vi "JSON Minify.vi"(8 "error in":errorcluster, 10 "JSON String":string) -> (0 "error out":errorcluster, 2 "JSON Minified":string)   [LabVIEW 2020]
doc: "This VI allows minifying the JSON prior to parsing to avoid any errors.\nThe algorithm is ported from https://github.com/getify/JSON.minify.\n---\nAuthor: Felipe P. Silva"
uses:
  <vilib>/regexp/Match Regular Expression.xnode
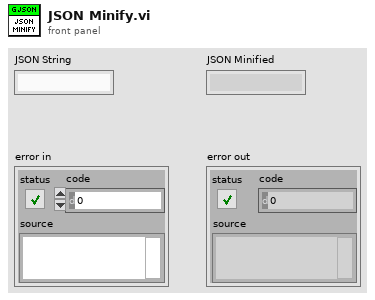
[diagram p1: front panel]
types:
  T1 = cluster{"in_multiline_comment":bool, "in_singleline_comment":bool, "in_string":bool, "new_str":string[], "from":i32, "lc":string, "rc":string}
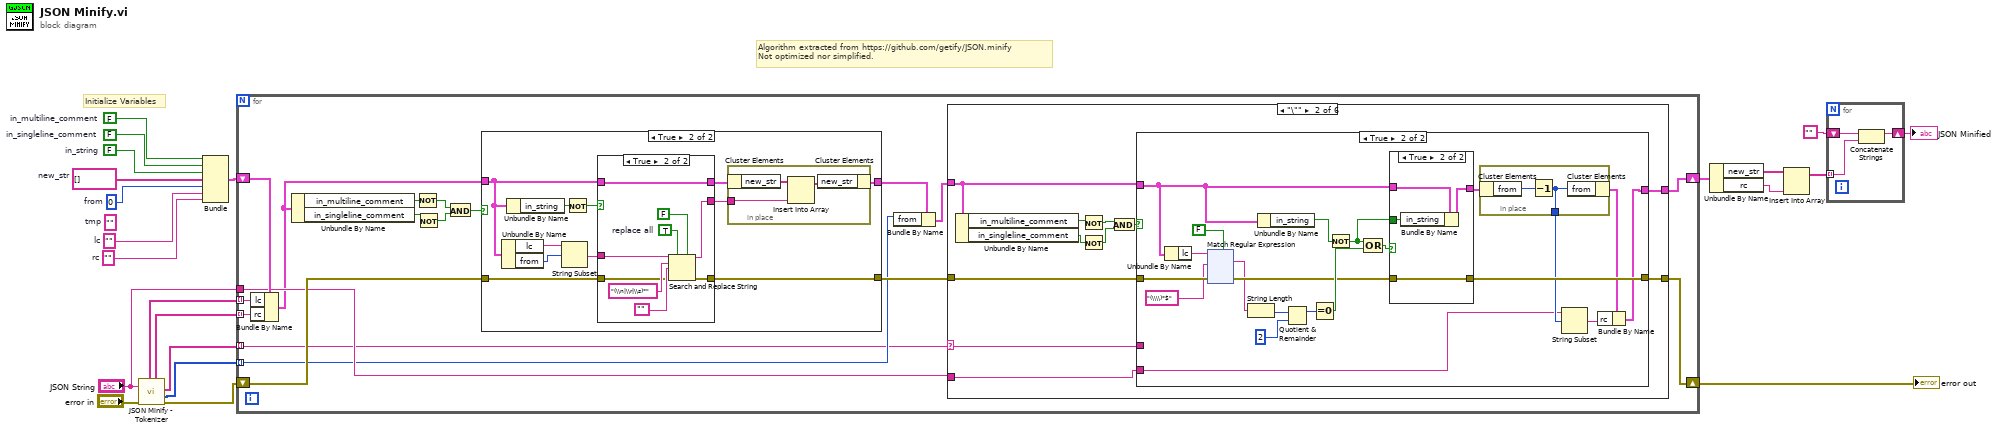
[diagram p0: block diagram]
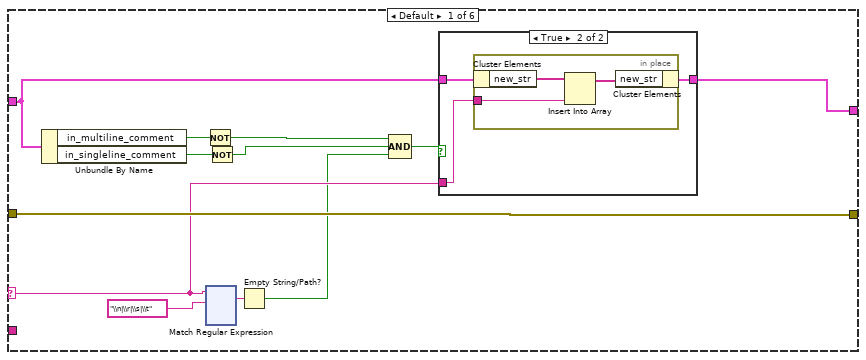
[diagram p2: hidden frame]
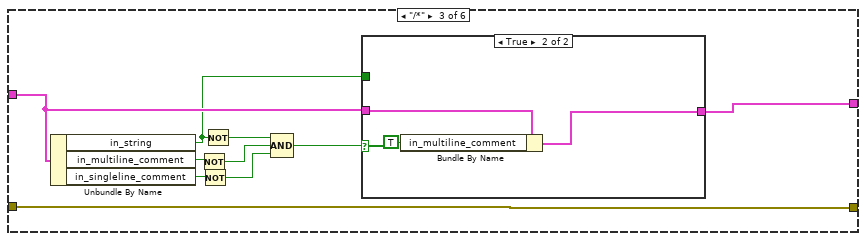
[diagram p6: hidden frame]
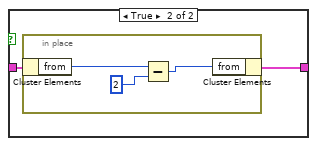
[diagram p8: hidden frame]
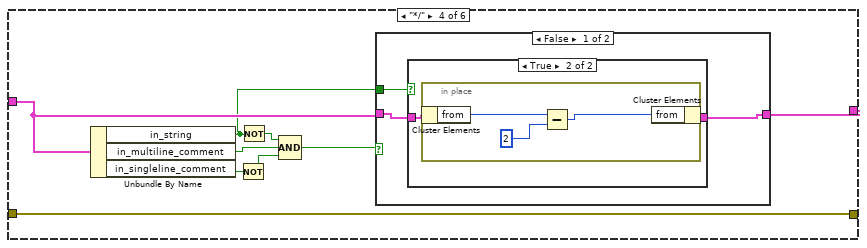
[diagram p9: hidden frame]
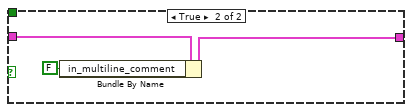
[diagram p11: hidden frame]
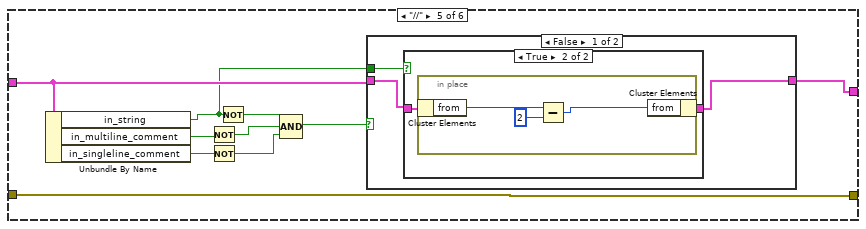
[diagram p12: hidden frame]
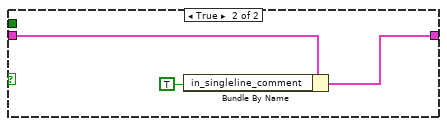
[diagram p14: hidden frame]
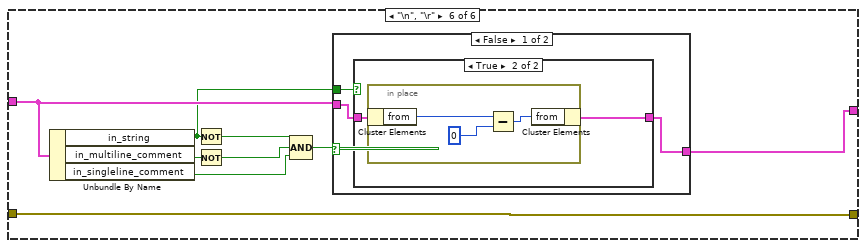
[diagram p15: hidden frame]
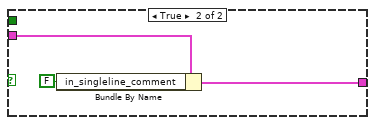
[diagram p17: hidden frame]
diagram:
  w12 = ""  # rc
  w13 = ""  # lc
  (unwired) ""  # tmp
  w19 = string[] []  # new_str
  w20 = FALSE  # in_string
  w21 = FALSE  # in_singleline_comment
  w22 = FALSE  # in_multiline_comment
  w17 = 0  # from
  # "Algorithm extracted from https://github.com/getify/JSON.minify\nNot optimized nor simplified."
  # "Initialize Variables"
  n1 = call "JSON Minify - Tokenizer.vi"("error in (no error)"="error in", "JSON String"="JSON String") -> ("error out"=w6:errorcluster, "offset past"=w5:i32[], "matches"=w4:string[], "Right Context"=w2:string[], "Left Context"=w3:string[])  [unwired: 5 in]
  n2 = Bundle("in_multiline_comment"=w22, "in_singleline_comment"=w21, "in_string"=w20, "new_str"=w19, "from"=w17, "lc"=w13, "rc"=w12) -> (w16:T1)  [unwired: 1 in]
  n3 = for {
    shift-right: [w29] -> w18
    shift-left: w6 -> [w35]
    shift-right: [w28] -> w11
    shift-left: w16 -> [w36]
    tunnel: w4 -> [w26] mode=indexing
    tunnel: "JSON String" -> [w32]
    tunnel: w5 -> [w27] mode=indexing
    tunnel: w3 -> [w24] mode=indexing
    tunnel: w2 -> [w23] mode=indexing
    n4 = Bundle By Name(cluster=w36, "lc"=w24, "rc"=w23) -> (w25:T1)
    n5 = Unbundle By Name(w25) -> ("in_multiline_comment"=w31:bool, "in_singleline_comment"=w30:bool)
    n6 = Not(x=w31) -> (.not. x?=w40:bool)
    n7 = Not(x=w30) -> (.not. x?=w39:bool)
    n8 = And(x=w40, y=w39) -> (x .and. y?=w37:bool)
    n9 = case shown="True" w37 {
      tunnel: w25 -> [w417 w421]
      tunnel: [w417 w425] -> w34
      tunnel: [w416 w428] -> w38
      tunnel: w35 -> [w416 w418]
      frame False {
      }
      frame True {
        n10 = Unbundle By Name(w421) -> ("lc"=w424:string, "from"=w423:i32)
        n11 = Unbundle By Name(w421) -> ("in_string"=w420:bool)
        n12 = String Subset(string=w424, offset (0)=w423) -> (substring=w422:string)  [unwired: 1 in]
        n13 = Not(x=w420) -> (.not. x?=w419:bool)
        n14 = case shown="True" w419 {
          tunnel: [w433 w443] -> w428
          tunnel: w421 -> [w434 w440]
          tunnel: [w434 w440] -> w426
          tunnel: [w432 w441] -> w427
          tunnel: w422 -> [w432 w438]
          tunnel: w418 -> [w433 w437]
          frame False {
          }
          frame True {
            w436 = TRUE  # replace all
            n15 = Search and Replace String(replace all?=w436, multiline?=FALSE ("multiline? (F)"), input string=w438, search string="(\\n|\\r|\\s)*", replace string="" ("replace string (\"\")"), error in=w437) -> (result string=w441:string, error out=w443:errorcluster)  [unwired: 2 in, 2 out]
          }
        }
        n16 = in-place {
          in-place-border: w427 -> [w430]
          n17 = in-place-cluster #1(w426) -> ("new_str"=w429:string[])
          n18 = Insert Into Array(array=w429, new element=w430) -> (w431:string[])  [unwired: 1 in]
          n19 = in-place-cluster #1("new_str"=w431) -> (w425:T1)
        }
      }
    }
    n20 = Bundle By Name(cluster=w34, "from"=w27) -> (w33:T1)
    n21 = case shown="\"\\\"\"" w26 {
      selector: w26 -> [w42 w175 _ _ _ _]
      tunnel: w33 -> [w51 w180 w338 w359 w381 w402]
      tunnel: [w50 w174 w336 w358 w380 w401] -> w28
      tunnel: w38 -> [w52 w183 w339 w360 w382 w403]
      tunnel: [w52 w184 w339 w360 w382 w403] -> w29
      tunnel: w32 -> [_ w176 _ _ _ _]
      frame Default {
        n22 = Unbundle By Name(w51) -> ("in_multiline_comment"=w46:bool, "in_singleline_comment"=w45:bool)
        n23 = Not(x=w46) -> (.not. x?=w49:bool)
        n24 = xnode "Match Regular Expression"("input string"=w42, "regular expression"="\\n|\\r|\\s|\\t") -> ("whole match"=w43:string)  [unwired: 4 in, 4 out]
        n25 = Not(x=w45) -> (.not. x?=w48:bool)
        n26 = Empty String/Path?(string/path=w43) -> (empty?=w41:bool)
        n27 = Compound Arithmetic op=AND(w49, w48, w41) -> (w47:bool)
        n28 = case shown="True" w47 {
          tunnel: w51 -> [w53 w56]
          tunnel: [w53 w55] -> w50
          tunnel: w42 -> [_ w54]
          frame False {
          }
          frame True {
            n29 = in-place {
              in-place-border: w54 -> [w57]
              n30 = in-place-cluster #2(w56) -> ("new_str"=w58:string[])
              n31 = Insert Into Array(array=w58, new element=w57) -> (w59:string[])  [unwired: 1 in]
              n32 = in-place-cluster #2("new_str"=w59) -> (w55:T1)
            }
          }
        }
      }
      frame "\"" {
        n33 = Unbundle By Name(w180) -> ("in_multiline_comment"=w178:bool, "in_singleline_comment"=w177:bool)
        n34 = Not(x=w178) -> (.not. x?=w181:bool)
        n35 = Not(x=w177) -> (.not. x?=w182:bool)
        n36 = And(x=w181, y=w182) -> (x .and. y?=w179:bool)
        n37 = case shown="True" w179 {
          tunnel: [w185 w207] -> w184
          tunnel: w183 -> [w185 w194]
          tunnel: [w186 w198] -> w174
          tunnel: w180 -> [w186 w199]
          tunnel: w176 -> [_ w196]
          tunnel: w175 -> [_ _]
          frame False {
          }
          frame True {
            n38 = Unbundle By Name(w199) -> ("lc"=w192:string)
            n39 = xnode "Match Regular Expression"("input string"=w192, "regular expression"="(\\\\)*$", "error in"=w194, "multiline? (F)"=FALSE) -> ("whole match"=w189:string, "error out"=w193:errorcluster)  [unwired: 2 in, 3 out]
            n40 = String Length(string=w189) -> (length=w190:i32)
            n41 = Unbundle By Name(w199) -> ("in_string"=w201:bool)
            n42 = Quotient & Remainder(x=w190, y=2) -> (x-y*floor(x/y)=w187:i32)  [unwired: 1 out]
            n43 = Equal To 0?(x=w187) -> (x = 0?=w202:bool)
            n44 = Not(x=w201) -> (.not. x?=w204:bool)
            n45 = Compound Arithmetic op=OR(w204, w202) -> (w205:bool)
            n46 = case shown="True" w205 {
              tunnel: [w210 w215] -> w207
              tunnel: w193 -> [w210 w215]
              tunnel: [w211 w213] -> w206
              tunnel: w199 -> [w211 w214]
              tunnel: w204 -> [_ w212]
              frame False {
              }
              frame True {
                n47 = Bundle By Name(cluster=w214, "in_string"=w212) -> (w213:T1)
              }
            }
            n48 = in-place {
              in-place-border: [w208] -> w197
              n49 = in-place-cluster #3(w206) -> ("from"=w209:i32)
              n50 = Decrement(x=w209) -> (x-1=w208:i32)
              n51 = in-place-cluster #3("from"=w208) -> (w200:T1)
            }
            n52 = String Subset(string=w196, offset (0)=w197) -> (substring=w195:string)  [unwired: 1 in]
            n53 = Bundle By Name(cluster=w200, "rc"=w195) -> (w198:T1)
          }
        }
      }
      frame "/*" {
        n54 = Unbundle By Name(w338) -> ("in_string"=w330:bool, "in_multiline_comment"=w335:bool, "in_singleline_comment"=w334:bool)
        n55 = Not(x=w335) -> (.not. x?=w332:bool)
        n56 = Not(x=w334) -> (.not. x?=w333:bool)
        n57 = Not(x=w330) -> (.not. x?=w331:bool)
        n58 = Compound Arithmetic op=AND(w331, w332, w333) -> (w337:bool)
        n59 = case shown="True" w337 {
          tunnel: w338 -> [w342 w351]
          tunnel: [w341 w350] -> w336
          tunnel: w330 -> [w340 _]
          frame False {
            n60 = case shown="False" w340 {
              tunnel: w342 -> [w343 w345]
              tunnel: [w343 w344] -> w341
              frame False {
              }
              frame True {
                n61 = in-place {
                  n62 = in-place-cluster #4(w345) -> ("from"=w348:i32)
                  n63 = Subtract(x=w348, y=2) -> (x-y=w347:i32)
                  n64 = in-place-cluster #4("from"=w347) -> (w344:T1)
                }
              }
            }
          }
          frame True {
            n65 = Bundle By Name(cluster=w351, "in_multiline_comment"=TRUE) -> (w350:T1)
          }
        }
      }
      frame "*/" {
        n66 = Unbundle By Name(w359) -> ("in_string"=w352:bool, "in_multiline_comment"=w354:bool, "in_singleline_comment"=w353:bool)
        n67 = Not(x=w353) -> (.not. x?=w356:bool)
        n68 = Not(x=w352) -> (.not. x?=w357:bool)
        n69 = Compound Arithmetic op=AND(w357, w354, w356) -> (w355:bool)
        n70 = case shown="False" w355 {
          tunnel: w359 -> [w363 w372]
          tunnel: [w362 w371] -> w358
          tunnel: w352 -> [w361 _]
          frame False {
            n71 = case shown="True" w361 {
              tunnel: w363 -> [w364 w366]
              tunnel: [w364 w365] -> w362
              frame False {
              }
              frame True {
                n72 = in-place {
                  n73 = in-place-cluster #5(w366) -> ("from"=w369:i32)
                  n74 = Subtract(x=w369, y=2) -> (x-y=w368:i32)
                  n75 = in-place-cluster #5("from"=w368) -> (w365:T1)
                }
              }
            }
          }
          frame True {
            n76 = Bundle By Name(cluster=w372, "in_multiline_comment"=FALSE) -> (w371:T1)
          }
        }
      }
      frame "//" {
        n77 = Unbundle By Name(w381) -> ("in_string"=w373:bool, "in_multiline_comment"=w375:bool, "in_singleline_comment"=w374:bool)
        n78 = Not(x=w375) -> (.not. x?=w378:bool)
        n79 = Not(x=w374) -> (.not. x?=w377:bool)
        n80 = Not(x=w373) -> (.not. x?=w379:bool)
        n81 = Compound Arithmetic op=AND(w379, w378, w377) -> (w376:bool)
        n82 = case shown="False" w376 {
          tunnel: w381 -> [w385 w394]
          tunnel: [w383 w393] -> w380
          tunnel: w373 -> [w384 _]
          frame False {
            n83 = case shown="True" w384 {
              tunnel: w385 -> [w386 w388]
              tunnel: [w386 w387] -> w383
              frame False {
              }
              frame True {
                n84 = in-place {
                  n85 = in-place-cluster #6(w388) -> ("from"=w391:i32)
                  n86 = Subtract(x=w391, y=2) -> (x-y=w390:i32)
                  n87 = in-place-cluster #6("from"=w390) -> (w387:T1)
                }
              }
            }
          }
          frame True {
            n88 = Bundle By Name(cluster=w394, "in_singleline_comment"=TRUE) -> (w393:T1)
          }
        }
      }
      frame "\n", "\r" {
        n89 = Unbundle By Name(w402) -> ("in_string"=w395:bool, "in_multiline_comment"=w398:bool, "in_singleline_comment"=w396:bool)
        n90 = Not(x=w395) -> (.not. x?=w400:bool)
        n91 = Not(x=w398) -> (.not. x?=w397:bool)
        n92 = Compound Arithmetic op=AND(w400, w397, w396) -> (w399:bool)
        n93 = case shown="False" w399 {
          tunnel: w402 -> [w406 w415]
          tunnel: [w405 w414] -> w401
          tunnel: w395 -> [w404 _]
          frame False {
            n94 = case shown="True" w404 {
              tunnel: w406 -> [w407 w409]
              tunnel: [w407 w408] -> w405
              frame False {
              }
              frame True {
                n95 = in-place {
                  n96 = in-place-cluster #7(w409) -> ("from"=w412:i32)
                  n97 = Subtract(x=w412, y=0) -> (x-y=w411:i32)
                  n98 = in-place-cluster #7("from"=w411) -> (w408:T1)
                }
              }
            }
          }
          frame True {
            n99 = Bundle By Name(cluster=w415, "in_singleline_comment"=FALSE) -> (w414:T1)
          }
        }
      }
    }
  }
  "error out" <- w18
  n100 = Unbundle By Name(w11) -> ("new_str"=w10:string[], "rc"=w9:string)
  n101 = Insert Into Array(array=w10, new element=w9) -> (w8:string[])  [unwired: 1 in]
  n102 = for {
    tunnel: w8 -> [w445] mode=indexing
    shift-right: [w444] -> w14
    shift-left: "" -> [w446]
    n103 = Concatenate Strings(w446, w445) -> (w444:string)
  }
  "JSON Minified" <- w14
